vi "FRCts20_Backend_Competition_POST.vi"(6 "Message Attributes":T4, 8 "error in (no error)":errorcluster, 10 "Data":string, 11 "Engine_Refnums":T1) -> (0 "error out":errorcluster)   [LabVIEW 2013]
doc: "Adds a new competition. Called by the competition/division api, and expects a competition name, start date, and duration."
uses:
  Dependencies/Keyed Array/KeyedArray.ctl
  FRCts20_Backend_EngineRefnums.ctl
  INI_Accessor/FRCts20_Backend_INI Controller.lvclass
  Dependencies/AMC/_SubVIs/TypeDefs/Message Queue.ctl
  Dependencies/AMC/_SubVIs/TypeDefs/Message.ctl
  <vilib>/addons/database/Connection.llb/Conn ObjectReference.ctl
  FRCts20_Backend_FGVOperation.ctl
  FRCts20_Backend_API/FRCts20_Backend_API_Competition.ctl
  FRCts20_Backend_Engine.lvlib
  FRCts20_Backend_API/FRCts20_Backend_API.lvlib
  Dependencies/Keyed Array/Tools_KeyedArray.lvlib
  Dependencies/AMC/AMC.lvlib
  <vilib>/addons/database/NI_Database_API.lvlib
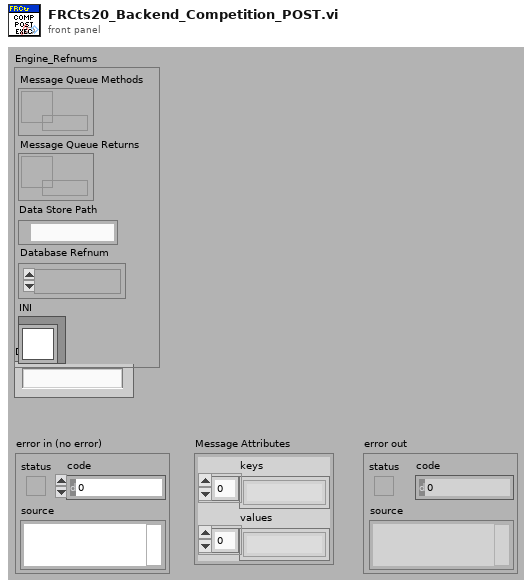
[diagram p1: front panel]
types:
  T1 = typedef "FRCts20_Backend_Engine.lvlib/FRCts20_Backend_EngineRefnums.ctl" = cluster{"Message Queue Methods":T2, "Message Queue Returns":T2, "Data Store Path":path, "Database Refnum":T3, "INI":refnum<class "FRCts20_Backend_INI Controller.lvclass">}
  T2 = typedef "AMC.lvlib/Message Queue.ctl" = refnum<queue>
  T3 = typedef "NI_Database_API.lvlib/Conn ObjectReference.ctl" = refnum<k1>
  T4 = typedef "Tools_KeyedArray.lvlib/KeyedArray.ctl" = cluster{"keys":string[], "values":string[]}
  T5 = typedef "FRCts20_Backend_API.lvlib/FRCts20_Backend_API_Competition.ctl" = cluster{"Name":string, "Start Date":timestamp, "Duration":u8, "Divisions":string[], "APIReturn":string}
  T6 = typedef "FRCts20_Backend_Engine.lvlib/FRCts20_Backend_FGVOperation.ctl" = enum16{"Initialize", "EnqueueMessage", "EnqueueDataReturn", "FlushMessage", "FlushDataReturn"}
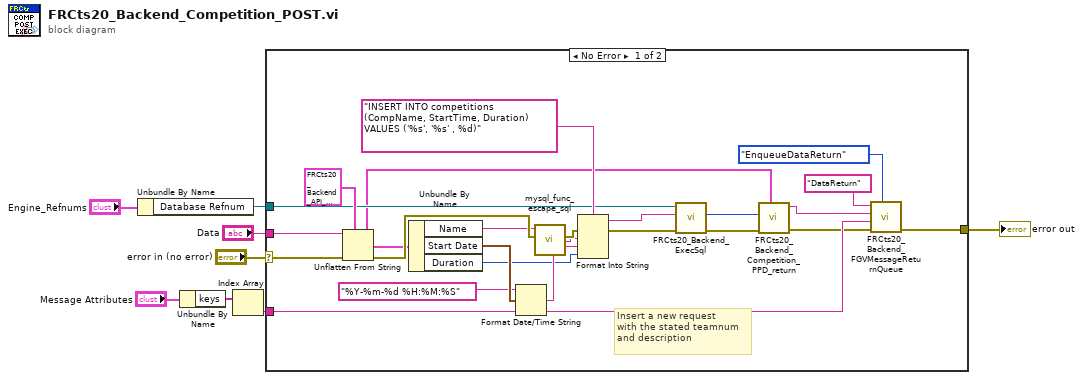
[diagram p0: block diagram]
diagram:
  n1 = Unbundle By Name("Engine_Refnums") -> ("Database Refnum"=w5:T3)
  n2 = Unbundle By Name("Message Attributes") -> ("keys"=w2:string[])
  n3 = Index Array(array=w2) -> (element=w1:string)  [unwired: 1 in]
  n4 = case shown="No Error" "error in (no error)" {
    selector: "error in (no error)" -> [w29 w33]
    tunnel: [w32 w33] -> w7
    tunnel: w5 -> [w16 _]
    tunnel: "Data" -> [w30 _]
    tunnel: w1 -> [w31 _]
    frame No Error {
      # "Insert a new request\nwith the stated teamnum\nand description"
      n5 = Unflatten From String(type=T5 {"Name"="", "Start Date"=timestamp(0 s since 1904-01-01), "Duration"=0, "Divisions"=[], "APIReturn"=""} ("Competition"), binary string=w30, error in (no error)=w29) -> (value=w13:T5, error out=w20:errorcluster)  [unwired: 2 in, 1 out]
      n6 = Unbundle By Name(w13) -> ("Name"=w19:string, "Start Date"=w24:timestamp, "Duration"=w21:u8)
      n7 = Format Date/Time String(time format string (%c)="%Y-%m-%d %H:%M:%S", seconds (now)=w24) -> (date/time string=w22:string)  [unwired: 1 in]
      n8 = call "mysql_func_escape_sql.vi"("error in (no error)"=w20, "sqlin"=w19) -> ("error out"=w18:errorcluster, "escaped"=w17:string)  [unwired: 8 in]
      n9 = Format Into String(format string="INSERT INTO competitions (CompName, StartTime, Duration) VALUES ('%s', '%s' , %d)", error in=w18, w17, w22, w21) -> (resulting string=w15:string, error out=w14:errorcluster)  [unwired: 1 in]
      n10 = call "FRCts20_Backend_ExecSql.vi"("error in (no error)"=w14, "format string"=w15, "Refnum in"=w16) -> ("error out"=w11:errorcluster, "rows affected"=w12:i32)  [unwired: 6 in, 1 out]
      n11 = call "FRCts20_Backend_Competition_PPD_return.vi"("Competition"=w13, "error in (no error)"=w11, "rows affected"=w12) -> ("error out"=w10:errorcluster, "data string"=w9:string)  [unwired: 7 in]
      n12 = call "FRCts20_Backend_FGVMessageReturnQueue.vi"("Operation"=FRCts20_Backend_FGVOperation."EnqueueDataReturn", "error in (no error)"=w10, "Key"=w31, "Message Value"=w9, "Message Name"="DataReturn") -> ("error out"=w32:errorcluster)  [unwired: 5 in, 1 out]
    }
    frame Error {
    }
  }
  "error out" <- w7
